vi "AssertSubpanelVIExecCore.vi"(0 "VI Reference In":refnum<vi>, 1 "Label":string, 2 "delimiter (>>)":string=">>", 3 "Assert Only? (F)":bool, 5 "Control Path":string, 7 "Execution:State":T2(array[ring]), 11 "Error In":errorcluster, 12 "Assert Interval(10 ms)":u32=10, 13 "Timeout(5 sec)":dbl=5.0) -> (4 "VI Reference Out":refnum<vi>, 6 "Asserted Value":T1(ring), 15 "Error Out":errorcluster)   [LabVIEW 2016, in "Drona.lvlib" / "AssertControlValue.lvlib" / "AssertSubpanel.lvlib"]
doc: "Asserts the execution state of Inserted VI in Subpanel.\n\nThe input control name is given as a string , incase of path, use delimiters inbetween the path."
uses:
  AssertSubpanel.lvlib
  Get/GetControlRef/GetControlRefByPath.vi
  <vilib>/addons/_JKI Toolkits/Caraya/classes/Assert/Assert True.vi
  <vilib>/addons/_JKI Toolkits/Caraya/classes/Assert/Assert.lvclass
  Get/GetControlRef/GetControlRef.lvlib
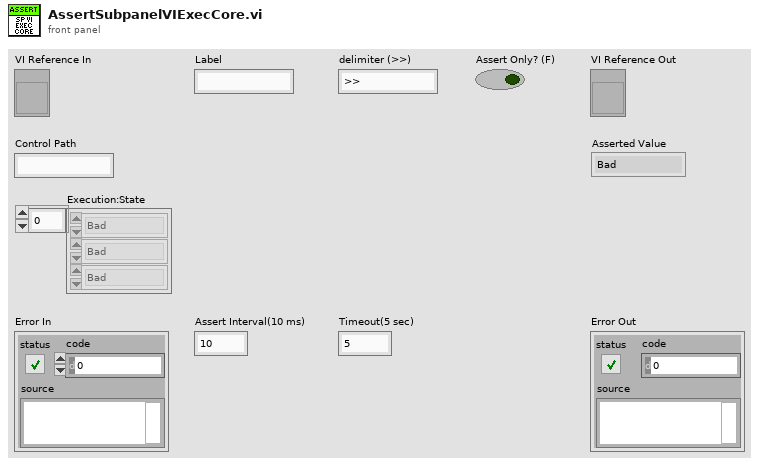
[diagram p1: front panel]
types:
  T1 = enum32{"Bad", "Idle", "Run top level", "Running"}
  T2 = enum32{"Bad", "Idle", "Run top level", "Running"}[]
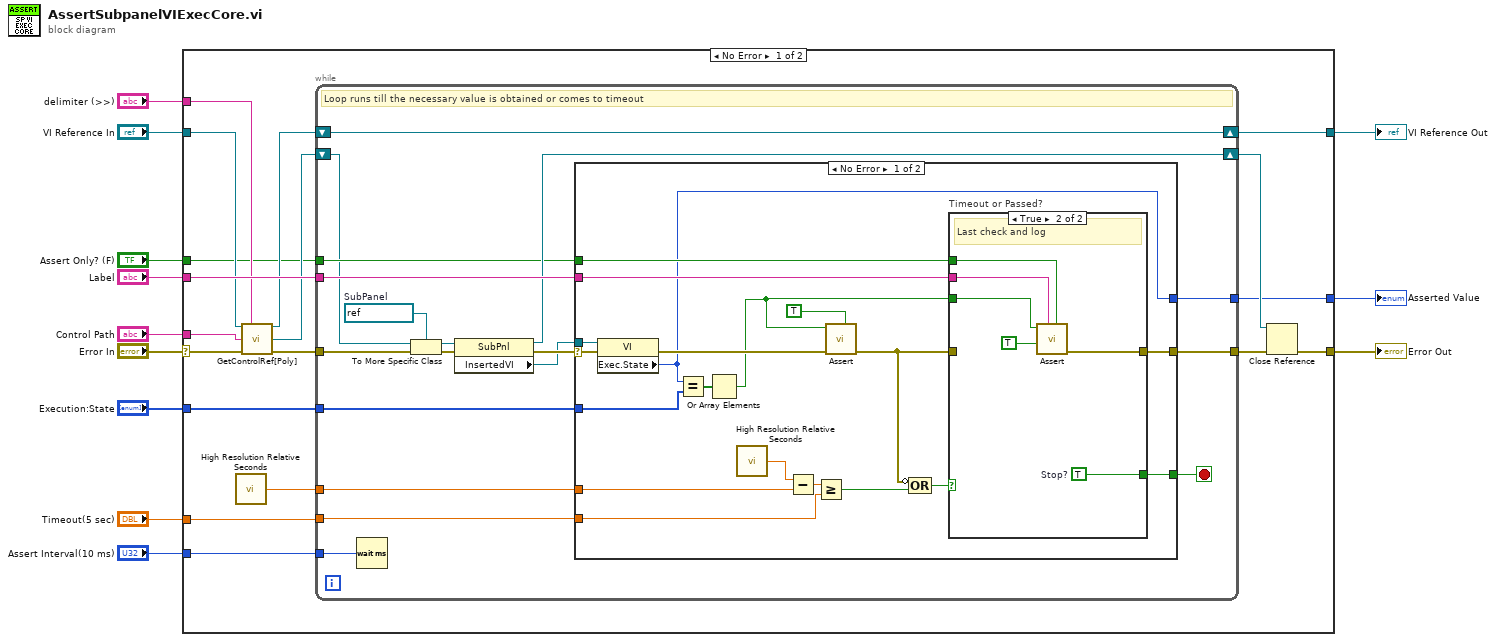
[diagram p0: block diagram]
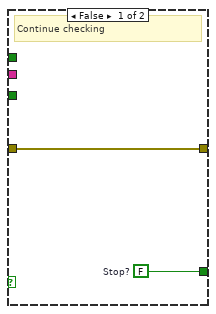
[diagram p2: hidden frame]
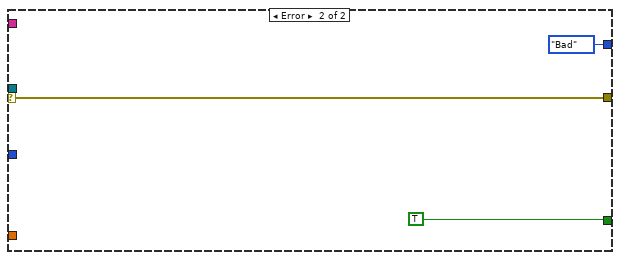
[diagram p3: hidden frame]
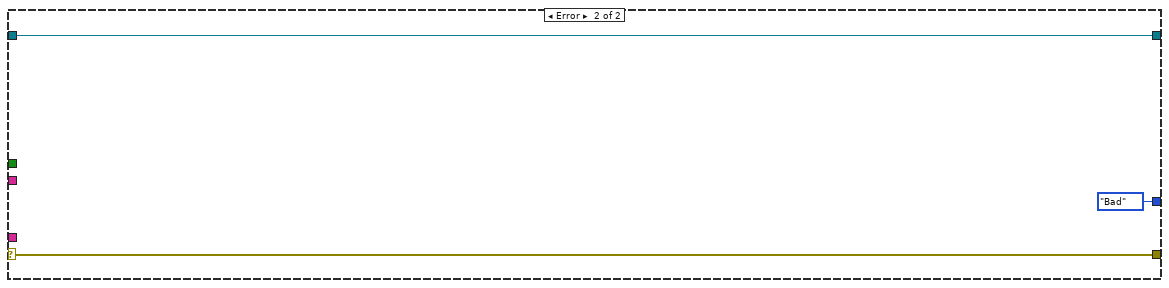
[diagram p4: hidden frame]
diagram:
  n1 = case shown="No Error" "Error In" {
    selector: "Error In" -> [w25 w81]
    tunnel: "Timeout(5 sec)" -> [w30 _]
    tunnel: [w29 w80] -> w11
    tunnel: [w18 w81] -> w10
    tunnel: "Assert Interval(10 ms)" -> [w27 _]
    tunnel: "Label" -> [w26 _]
    tunnel: "VI Reference In" -> [w24 w80]
    tunnel: "Control Path" -> [w23 _]
    tunnel: "delimiter (>>)" -> [w16 _]
    tunnel: "Assert Only? (F)" -> [w15 _]
    tunnel: "Execution:State" -> [w14 _]
    tunnel: [w13 T1."Bad" ("Exec.State")] -> w1
    frame No Error {
      n2 = call <vilib>:"High Resolution Relative Seconds.vi"() -> ("relative seconds"=w22:dbl)
      n3 = call-poly "GetControlRef[Poly].vi"("VI Reference In"=w24, "delimiter (>>)"=w16, "Control Path"=w23, "error In"=w25) -> ("VI Reference Out"=w20:refnum<vi>, "Ctl Refnum"=w19:refnum<vi>, "error out"=w21:errorcluster)  [unwired: 9 in]
      n4 = while {
        tunnel: w30 -> [w47]
        tunnel: w22 -> [w48]
        tunnel: w21 -> [w42]
        tunnel: [w45] -> w28
        tunnel: w27 -> [w43]
        tunnel: w26 -> [w40]
        shift-right: [w41] -> w29
        shift-left: w20 -> [w41]
        shift-right: [w39] -> w17
        shift-left: w19 -> [w33]
        tunnel: w15 -> [w38]
        tunnel: w14 -> [w36]
        tunnel: [w31] -> w13
        stop <- w46 stop-if-true
        w34 = refnum<vi> refnum  # SubPanel
        # "Loop runs till the necessary value is obtained or comes to timeout"
        n5 = Wait (ms)(milliseconds to wait=w43) -> ()  [unwired: 1 out]
        n6 = To More Specific Class(target class=w34, reference=w33, error in=w42) -> (specific class reference=w32:refnum<vi>, error out=w35:errorcluster)
        n7 = property class="SubPnl"(reference=w32, error in=w35) -> (reference out=w39:refnum<vi>, error out=w44:errorcluster, "InsertedVI"=w37:refnum<vi>)
        n8 = case shown="No Error" w44 {
          selector: w44 -> [w54 w78]
          tunnel: w48 -> [w67 _]
          tunnel: w47 -> [w64 _]
          tunnel: [w57 TRUE] -> w46
          tunnel: [w58 w78] -> w45
          tunnel: w37 -> [w55 _]
          tunnel: w40 -> [w63 _]
          tunnel: w38 -> [w56 _]
          tunnel: w36 -> [w52 _]
          tunnel: [w49 T1."Bad" ("Exec.State")] -> w31
          frame No Error {
            n9 = property class="VI"(reference=w55, error in=w54) -> (error out=w53:errorcluster, "Exec.State"=w49:T1)  [unwired: 1 out]
            n10 = Equal?(x=w49, y=w52) -> (x = y?=w51:bool[])
            n11 = Or Array Elements(Boolean array=w51) -> (logical OR=w50:bool)
            n12 = call <vilib>:"High Resolution Relative Seconds.vi"() -> ("relative seconds"=w66:dbl)
            n13 = Subtract(x=w66, y=w67) -> (x-y=w65:dbl)
            n14 = Greater Or Equal?(x=w65, y=w64) -> (x >= y?=w62:bool)
            n15 = call-poly <vilib>:"Assert.vi"("Assert Only? (F)"=TRUE, "error in (no error)"=w53, "True?"=w50) -> ("error out"=w61:errorcluster)  [unwired: 7 in, 1 out]
            n16 = Compound Arithmetic op=OR(invert w61, w62) -> (w60:bool)
            n17 = case "Timeout or Passed?" shown="True" w60 {
              tunnel: w61 -> [w69 _]
              tunnel: w50 -> [_ w70]
              tunnel: w63 -> [_ w75]
              tunnel: [w69 w74] -> w58
              tunnel: [w68 w73] -> w57
              tunnel: w56 -> [_ w71]
              frame False {
                w68 = FALSE  # Stop?
                # "Continue checking"
              }
              frame True {
                w73 = TRUE  # Stop?
                # "Last check and log"
                n18 = call-poly <vilib>:"Assert.vi"("Assert Only? (F)"=w71, "Label"=w75, "Register with caller test (F)"=TRUE, "True?"=w70) -> ("error out"=w74:errorcluster)  [unwired: 6 in, 1 out]
              }
            }
          }
          frame Error {
          }
        }
      }
      n19 = Close Reference(reference=w17, error in (no error)=w28) -> (error out=w18:errorcluster)
    }
    frame Error {
    }
  }
  "Error Out" <- w10
  "VI Reference Out" <- w11
  "Asserted Value" <- w1
